vi "Silver--constant.vi"() -> (1 "Color":u32(colorbox)=12632256)   [LabVIEW 2018, in "Resistor Band Colors.lvlib"]
uses:
  Resistor Band Colors.lvlib
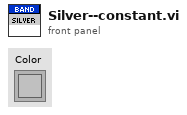
[diagram p1: front panel]
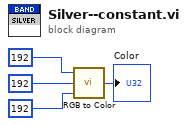
[diagram p0: block diagram]
diagram:
  n1 = call <vilib>:"RGB to Color.vi"("B"=u8 192, "G"=u8 192, "R"=u8 192) -> ("Color"=→"Color":u32)
